vi "Driving with the Limelight.vi"() -> (0 "TurnCommand":dbl(knob)=nan scale=-1.0..1.0, 1 "SpeedCommand":dbl(knob)=-0.0 scale=0.0..1.0, 3 "TargetValid":bool)   [LabVIEW 2019]
uses:
  Framework/Robot Global Data.vi
  <vilib>/addons/control/pid/NI_PID_pid.lvlib
  <vilib>/addons/control/pid/pid.llb/PID (DBL).vi
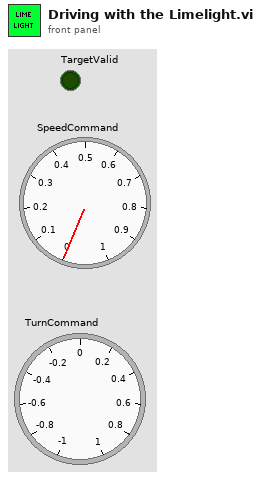
[diagram p1: front panel]
types:
  T1 = cluster{"proportional gain (Kc)":dbl, "integral time (Ti, min)":dbl, "derivative time (Td, min)":dbl}
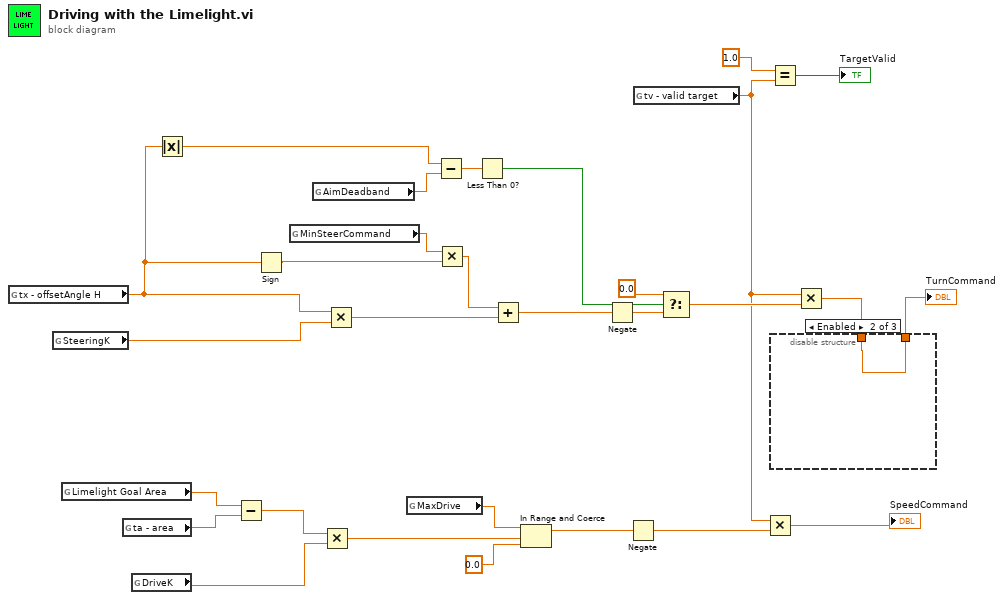
[diagram p0: block diagram]
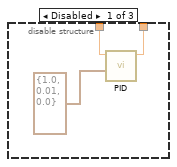
[diagram p2: hidden frame]
diagram:
  n1 = global read "Robot Global Data.vi" "tx - offsetAngle H"() -> (w12:dbl)
  n2 = global read "Robot Global Data.vi" "SteeringK"() -> (w6:dbl)
  n3 = global read "Robot Global Data.vi" "Limelight Goal Area"() -> (w7:dbl)
  n4 = global read "Robot Global Data.vi" "ta - area"() -> (w11:dbl)
  n5 = global read "Robot Global Data.vi" "DriveK"() -> (w8:dbl)
  n6 = Absolute Value(x=w12) -> (abs(x)=w26:dbl)
  n7 = Subtract(x=w7, y=w11) -> (x-y=w21:dbl)
  n8 = Sign(1:w12) -> (0:w22:dbl)
  n9 = global read "Robot Global Data.vi" "MinSteerCommand"() -> (w4:dbl)
  n10 = global read "Robot Global Data.vi" "AimDeadband"() -> (w5:dbl)
  n11 = Multiply(x=w21, y=w8) -> (x*y=w20:dbl)
  n12 = Multiply(x=w12, y=w6) -> (x*y=w24:dbl)
  n13 = global read "Robot Global Data.vi" "MaxDrive"() -> (w9:dbl)
  n14 = Subtract(x=w26, y=w5) -> (x-y=w27:dbl)
  n15 = Multiply(x=w4, y=w22) -> (x*y=w25:dbl)
  n16 = Less Than 0?(x=w27) -> (x < 0?=w28:bool)
  n17 = Add(x=w25, y=w24) -> (x+y=w15:dbl)
  n18 = In Range and Coerce(upper limit=w9, x=w20, lower limit=0.0) -> (coerced(x)=w17:dbl)  [unwired: 1 out]
  n19 = Negate(x=w15) -> (-x=w3:dbl)
  n20 = Negate(x=w17) -> (-x=w16:dbl)
  n21 = global read "Robot Global Data.vi" "tv - valid target"() -> (w10:dbl)
  n22 = Select(t=0.0, s=w28, f=w3) -> (s? t:f=w23:dbl)
  n23 = Multiply(x=w10, y=w16) -> (x*y=→"SpeedCommand":dbl)
  n24 = Equal?(x=1.0, y=w10) -> (x = y?=→"TargetValid":bool)
  n25 = Multiply(x=w10, y=w23) -> (x*y=w2:dbl)
  n26 = disable-structure shown="Enabled" {
    disable-tunnel: w2 -> [w32 w33 _]
    disable-tunnel: [w31 w33 _] -> w1
    frame Disabled {
      n27 = call-poly <vilib>:"PID.vi"("PID gains"=T1 {"proportional gain (Kc)"=1.0, "integral time (Ti, min)"=0.01, "derivative time (Td, min)"=0.0}, "setpoint"=w32) -> ("output"=w31:dbl)  [unwired: 8 in, 1 out]
    }
    frame Enabled {
    }
    frame Disabled {
    }
  }
  "TurnCommand" <- w1
